vi "Configure Volume Correction.vi"(7 "Pump ID (0:A)":T1, 8 "error in (no error)":errorcluster, 10 "Calibration Factor (1.0)":dbl=1.0, 11 "VISA resource in":refnum<visa-resource-name>) -> (0 "error out":errorcluster, 3 "VISA resource out":refnum<visa-resource-name>)   [LabVIEW 2015, in "Global FIA milliGAT.lvlib"]
doc: "Configuration the motion settings:; initial flow rate, acceleration, deceleration, and max flow rate."
uses:
  Global FIA milliGAT.lvlib
  Private/Pump Parameter.ctl
  Utility/Pump Address.ctl
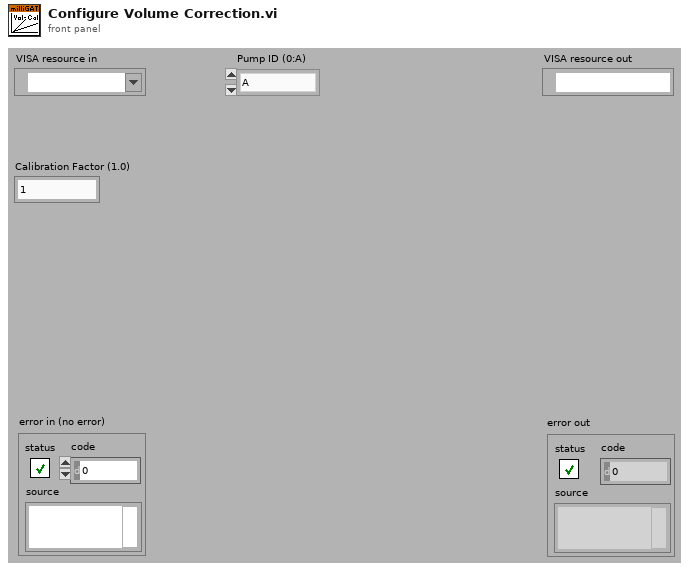
[diagram p1: front panel]
types:
  T1 = typedef "Global FIA milliGAT.lvlib/Pump Address.ctl" = enum16{"A", "B", "C", "D", "E", "F", "G", "H", "I", "J", "K", "L", "M", "N", "O", "P", "Q", "R", "S", "T", "U", "V", "W", "X", "Y", "Z", "a", "b", "c", "d", "e", "f", "g", "h", "i", "j", "k", "l", "m", "n", "o", "p", "q", "r", "s", "t", "u", "v", "w", "x", "y", "z", "0", "1", "2", "3", "4", "5", "6", "7", "8", "9"}
  T2 = typedef "Global FIA milliGAT.lvlib/Pump Parameter.ctl" = enum16{"Enabled", "EU", "EU Calibration Factor", "Fixed Asp or Disp", "Starting Position", "Starting Flow", "Peak Flow", "Flow Acceleration", "Flow Deceleration", "Session Volume", "Max Pressure", "Backlash (usteps)", "BL Calibration Factor", "BL Correction Enabled", "Min Flow", "Max Flow", "Min Acceleration", "Max Acceleration", "Service Volume", "Life Volume"}
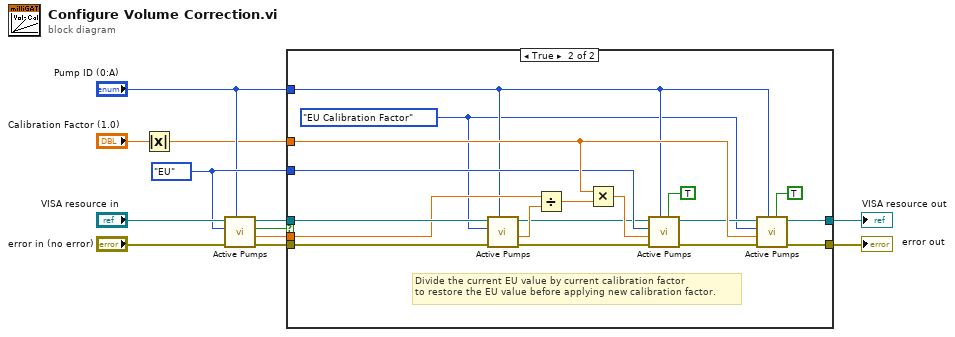
[diagram p0: block diagram]
diagram:
  w4 = Pump_Parameter."EU" ("Parameter")
  n1 = Absolute Value(x="Calibration Factor (1.0)") -> (abs(x)=w1:dbl)
  n2 = call "Active Pumps.vi"("Pump ID (0:A)"="Pump ID (0:A)", "error in (no error)"="error in (no error)", "Parameter"=w4, "VISA resource in"="VISA resource in") -> ("error out"=w8:errorcluster, "Value out"=w9:dbl, "Found"=w3:bool, "VISA resource out"=w7:refnum<visa-resource-name>)  [unwired: 4 in]
  n3 = case shown="True" w3 {
    tunnel: [w14 w32] -> w12
    tunnel: [w13 w31] -> w11
    tunnel: "Pump ID (0:A)" -> [_ w16]
    tunnel: w1 -> [_ w29]
    tunnel: w9 -> [_ w20]
    tunnel: w8 -> [w14 w23]
    tunnel: w7 -> [w13 w22]
    tunnel: w4 -> [_ w25]
    frame False {
      # "Not Found"
    }
    frame True {
      w15 = Pump_Parameter."EU Calibration Factor" ("Parameter")
      # "Divide the current EU value by current calibration factor\nto restore the EU value before applying new calibration factor."
      n4 = call "Active Pumps.vi"("Pump ID (0:A)"=w16, "error in (no error)"=w23, "Parameter"=w15, "VISA resource in"=w22) -> ("error out"=w18:errorcluster, "Value out"=w19:dbl, "VISA resource out"=w17:refnum<visa-resource-name>)  [unwired: 4 in, 1 out]
      n5 = Divide(x=w20, y=w19) -> (x/y=w21:dbl)
      n6 = Multiply(x=w29, y=w21) -> (x*y=w26:dbl)
      n7 = call "Active Pumps.vi"("Action (F:Read)"=TRUE, "Pump ID (0:A)"=w16, "error in (no error)"=w18, "Value in"=w26, "Parameter"=w25, "VISA resource in"=w17) -> ("error out"=w28:errorcluster, "VISA resource out"=w27:refnum<visa-resource-name>)  [unwired: 2 in, 2 out]
      n8 = call "Active Pumps.vi"("Action (F:Read)"=TRUE, "Pump ID (0:A)"=w16, "error in (no error)"=w28, "Value in"=w29, "Parameter"=w15, "VISA resource in"=w27) -> ("error out"=w32:errorcluster, "VISA resource out"=w31:refnum<visa-resource-name>)  [unwired: 2 in, 2 out]
    }
  }
  "VISA resource out" <- w11
  "error out" <- w12
